vi "3458A Read Digital Sample Memory.vi"(0 "VISA session":refnum<visa-resource-name>, 1 "read timeout [ms] (30000s)":u32=30000, 2 "display string (none)":string, 5 "First Read in Memory Location (0)":i32, 9 "max read [smpl]":i32=-1 caption="Max Read (-1: all)", 11 "error in (no error)":errorcluster) -> (3 "total samples in memory?":i32, 4 "dup VISA session":refnum<visa-resource-name>, 6 "waveform data [V]":dbl[](array[numeric]), 10 "waveform data int32":i32[](array[numeric]), 12 "read samples":i32, 14 "scale factor":dbl, 15 "error out":errorcluster)   [LabVIEW 2013, in "3458A Virtual Digitizer.lvlib" / "3458A Digitizing Low Levels.lvlib"]
doc: "Reads digitized data from memory. If 'Max Read' is set to -1 it reads all available data. It should work with SINt, DINT, SREAL and DREAL modes. ASCII read mode is not finished. It selects the OFORMAT automaticlaly. Data are returned already scaled if transfered in INT."
uses:
  3458A Digitizing Low Levels.lvlib
  3458A Basic Driver/3458A Basic Driver.lvlib
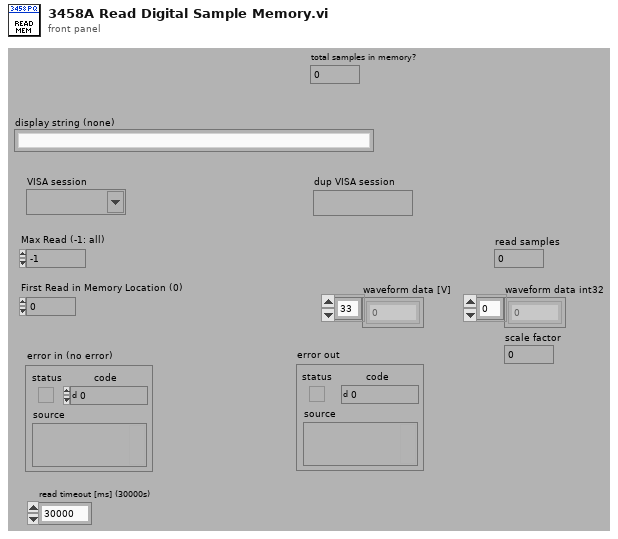
[diagram p1: front panel]
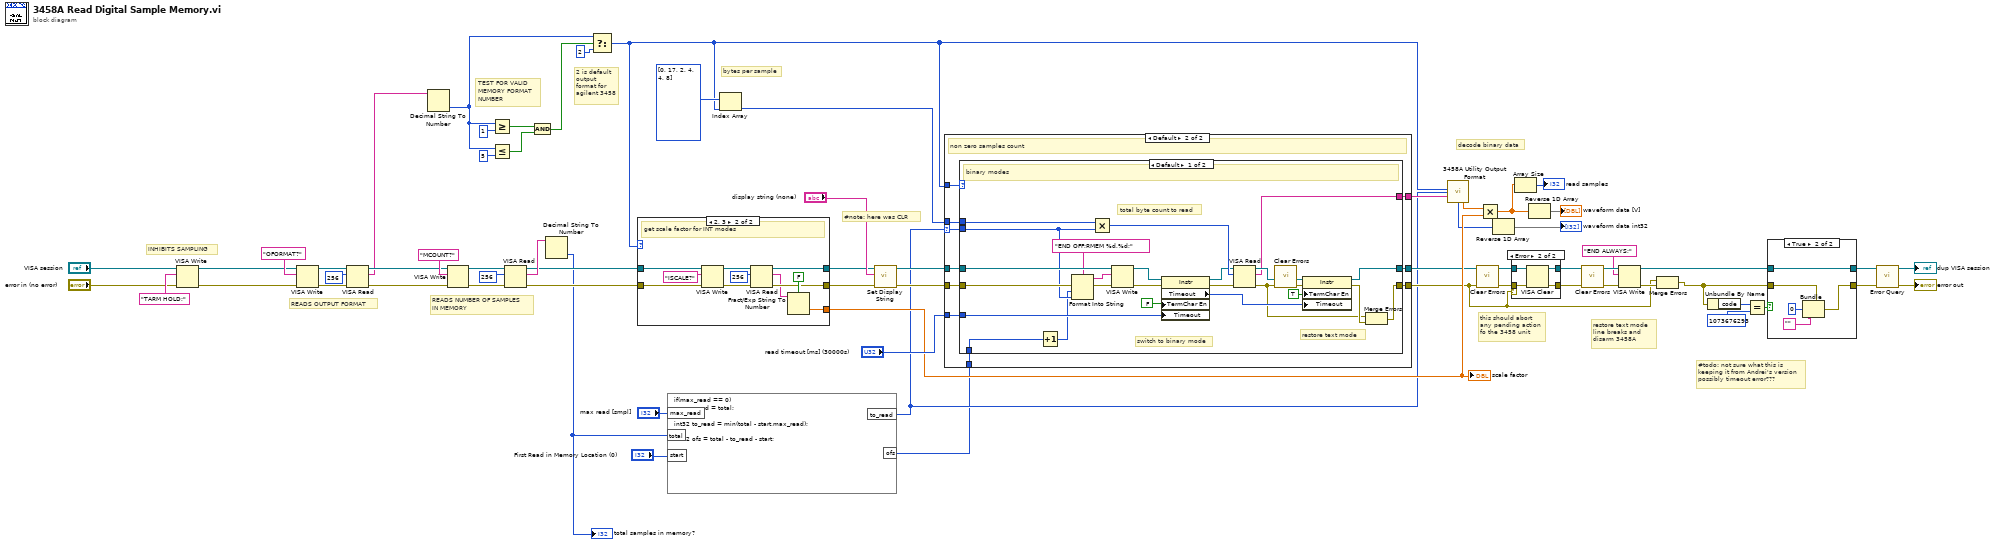
[diagram p0: block diagram]
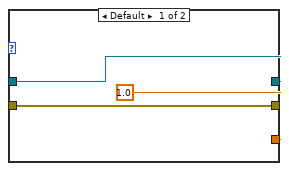
[diagram p5: hidden frame]
diagram:
  # "#note: here was CLR"
  # "restore text mode\nline breaks and\ndisarm 3458A"
  # "this should abort\nany pending action\nfo the 3458 unit"
  # "decode binary data"
  # "#todo: not sure what this is\nkeeping it from Andrei's version\npossibly timeout error???"
  # "bytes per sample"
  # "2 is default\noutput\nformat for\nagilent 3458"
  # "TEST FOR VALID\nMEMORY FORMAT\nNUMBER"
  # "READS NUMBER OF SAMPLES\nIN MEMORY"
  # "READS OUTPUT FORMAT"
  # "INHIBITS SAMPLING"
  n1 = VISA Write(VISA resource name="VISA session", write buffer="TARM HOLD;", error in (no error)="error in (no error)") -> (VISA resource name out=w31:refnum<visa-resource-name>, error out=w33:errorcluster)  [unwired: 1 out]
  n2 = VISA Write(VISA resource name=w31, write buffer="OFORMAT?", error in (no error)=w33) -> (VISA resource name out=w49:refnum<visa-resource-name>, error out=w48:errorcluster)  [unwired: 1 out]
  n3 = VISA Read(VISA resource name=w49, byte count=u32 256, error in (no error)=w48) -> (VISA resource name out=w47:refnum<visa-resource-name>, read buffer=w45:string, error out=w46:errorcluster)  [unwired: 1 out]
  n4 = Decimal String To Number(string=w45) -> (number=w39:i32)  [unwired: 2 in, 1 out]
  n5 = VISA Write(VISA resource name=w47, write buffer="MCOUNT?", error in (no error)=w46) -> (VISA resource name out=w56:refnum<visa-resource-name>, error out=w55:errorcluster)  [unwired: 1 out]
  n6 = Greater Or Equal?(x=w39, y=1) -> (x >= y?=w41:bool)
  n7 = Less Or Equal?(x=w39, y=5) -> (x <= y?=w42:bool)
  n8 = VISA Read(VISA resource name=w56, byte count=u32 256, error in (no error)=w55) -> (VISA resource name out=w52:refnum<visa-resource-name>, read buffer=w54:string, error out=w51:errorcluster)  [unwired: 1 out]
  n9 = And(x=w41, y=w42) -> (x .and. y?=w40:bool)
  n10 = Decimal String To Number(string=w54) -> (number=w3:i32)  [unwired: 2 in, 1 out]
  "total samples in memory?" <- w3
  n11 = Select(t=w39, s=w40, f=2) -> (s? t:f=w23:i32)
  n12 = case shown="2, 3" w23 {
    tunnel: [w67 w74] -> w5
    tunnel: [w68 w73] -> w4
    tunnel: w52 -> [w68 w72]
    tunnel: w51 -> [w67 w71]
    tunnel: [1.0 w69] -> w34
    frame Default {
    }
    frame 2, 3 {
      # "get scale factor for INT modes"
      n13 = VISA Write(VISA resource name=w72, write buffer="ISCALE?", error in (no error)=w71) -> (VISA resource name out=w77:refnum<visa-resource-name>, error out=w76:errorcluster)  [unwired: 1 out]
      n14 = VISA Read(VISA resource name=w77, byte count=u32 256, error in (no error)=w76) -> (VISA resource name out=w73:refnum<visa-resource-name>, read buffer=w70:string, error out=w74:errorcluster)  [unwired: 1 out]
      n15 = Fract/Exp String To Number(use system decimal point (T)=FALSE, string=w70) -> (number=w69:dbl)  [unwired: 2 in, 1 out]
    }
  }
  "scale factor" <- w34
  n16 = formula code="if(max_read == 0)\n  max_read = total;\n\nint32 to_read = min(total - start,max_read);\n\nint32 ofs = total - to_read - start;"("max_read"="max read [smpl]", "total"=w3, "start"="First Read in Memory Location (0)") -> ("to_read"=w6:i32, "ofs"=w2:i32)
  n17 = Index Array(array=i32[] [0, 17, 2, 4, 4, 8], index=w23) -> (element=w36:i32)
  n18 = call "Set Display String.vi"("error in(no error)"=w5, "display string (none)"="display string (none)", "VISA Resource Name"=w4) -> ("error out"=w11:errorcluster, "VISA resource name out"=w10:refnum<visa-resource-name>)  [unwired: 7 in]
  n19 = case shown="Default" w6 {
    selector: w6 -> [_ w83]
    tunnel: w10 -> [w80 w91]
    tunnel: w11 -> [w81 w90]
    tunnel: w36 -> [_ w89]
    tunnel: w23 -> [_ w88]
    tunnel: "read timeout [ms] (30000s)" -> [_ w87]
    tunnel: [w81 w86] -> w8
    tunnel: [w80 w85] -> w14
    tunnel: [_ w84] -> w30
    tunnel: w2 -> [_ w82]
    frame 0 {
    }
    frame Default {
      # "non zero samples count"
      n20 = case shown="Default" w88 {
        tunnel: w91 -> [w108 w118]
        tunnel: w90 -> [w103 w117]
        tunnel: w89 -> [w107 _]
        tunnel: w83 -> [w99 _]
        tunnel: [w93 w118] -> w85
        tunnel: [w96 w117] -> w86
        tunnel: [w106 _] -> w84
        tunnel: w87 -> [w101 _]
        tunnel: w82 -> [w92 _]
        frame Default {
          # "restore text mode"
          # "switch to binary mode"
          # "total byte count to read"
          # "binary modes"
          n21 = Increment(x=w92) -> (x+1=w98:i32)
          n22 = Format Into String(format string="END OFF;RMEM %d,%d;", error in=w103, w98, w99) -> (resulting string=w102:string, error out=w104:errorcluster)  [unwired: 1 in]
          n23 = Multiply(x=w107, y=w99) -> (x*y=w116:i32)
          n24 = VISA Write(VISA resource name=w108, write buffer=w102, error in (no error)=w104) -> (VISA resource name out=w114:refnum<visa-resource-name>, error out=w113:errorcluster)  [unwired: 1 out]
          n25 = property on="Property Node" class="Instr"(reference=w114, error in=w113, "TermChar En"=FALSE, "Timeout"=w101) -> (reference out=w112:refnum<visa-resource-name>, error out=w111:errorcluster, "Timeout"=w100:u32)
          n26 = VISA Read(VISA resource name=w112, byte count=w116, error in (no error)=w111) -> (VISA resource name out=w109:refnum<visa-resource-name>, read buffer=w106:string, error out=w95:errorcluster)  [unwired: 1 out]
          n27 = call <vilib>:"Clear Errors.vi"("error in (no error)"=w95) -> ("error out"=w94:errorcluster)  [unwired: 6 in]
          n28 = property class="Instr"(reference=w109, error in=w94, "TermChar En"=TRUE, "Timeout"=w100) -> (reference out=w93:refnum<visa-resource-name>, error out=w97:errorcluster)
          n29 = Merge Errors(w95, w97) -> (w96:errorcluster)
        }
        frame 1 {
          # "ASCII - not done"
        }
      }
    }
  }
  n30 = call "3458A Utility Output Format.vi"("Output Format (0:ASCII)"=w23, "Numbers of Reading (1)"=w6, "Input String"=w30) -> ("binary converted to int32"=w26:i32[], "anything converted to double"=w29:dbl[])  [unwired: 6 in, 5 out]
  n31 = call <vilib>:"Clear Errors.vi"("error in (no error)"=w8) -> ("error out"=w20:errorcluster)  [unwired: 6 in]
  n32 = Multiply(x=w29, y=w34) -> (x*y=w25:dbl[])
  n33 = Reverse 1D Array(array=w26) -> (reversed array=→"waveform data int32":i32[])
  n34 = case shown="Error" w8 {
    tunnel: w20 -> [w119 w124]
    tunnel: [w119 w123] -> w19
    tunnel: [w120 w122] -> w17
    tunnel: w14 -> [w120 w121]
    frame No Error {
    }
    frame Error {
      n35 = VISA Clear(VISA resource name=w121, error in (no error)=w124) -> (VISA resource name out=w122:refnum<visa-resource-name>, error out=w123:errorcluster)
    }
  }
  n36 = Array Size(array=w25) -> (size(s)=→"read samples":i32)
  n37 = Reverse 1D Array(array=w25) -> (reversed array=→"waveform data [V]":dbl[])
  n38 = call <vilib>:"Clear Errors.vi"("error in (no error)"=w19) -> ("error out"=w18:errorcluster)  [unwired: 6 in]
  n39 = VISA Write(VISA resource name=w17, write buffer="END ALWAYS;", error in (no error)=w18) -> (VISA resource name out=w12:refnum<visa-resource-name>, error out=w15:errorcluster)  [unwired: 1 out]
  n40 = Merge Errors(w8, w15) -> (w13:errorcluster)
  n41 = Unbundle By Name(w13) -> ("code"=w65:i32)
  n42 = Equal?(x=w65, y=1073676293 ("The specified termination character  was read")) -> (x = y?=w63:bool)
  n43 = case shown="True" w63 {
    tunnel: w13 -> [w126 w131]
    tunnel: [w126 w130] -> w61
    tunnel: [w125 w127] -> w62
    tunnel: w12 -> [w125 w127]
    frame False {
    }
    frame True {
      n44 = Bundle(cluster=w131, "code"=0, "source"="" ("Empty String")) -> (w130:errorcluster)  [unwired: 1 in]
    }
  }
  n45 = call "Error Query.vi"("error in (no error)"=w61, "VISA resource name"=w62) -> ("error out"=→"error out":errorcluster, "VISA resource name out"=→"dup VISA session":refnum<visa-resource-name>)  [unwired: 6 in, 2 out]
